vi "Disconnect Datastream Port.vi"(8 "error in (no error)":errorcluster, 11 "OXY_SCPI Reseource Out":refnum<visa-resource-name>) -> (0 "error out":errorcluster)   [LabVIEW 2020, in "OXYGEN_Datastream.lvlib"]
uses:
  OXYGEN_Datastream.lvlib
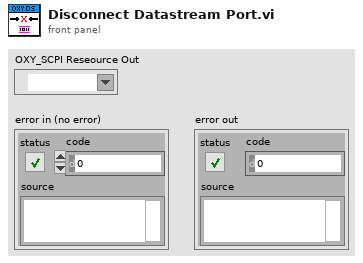
[diagram p1: front panel]
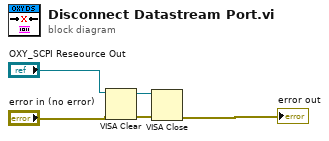
[diagram p0: block diagram]
diagram:
  n1 = VISA Clear(VISA resource name="OXY_SCPI Reseource Out", error in (no error)="error in (no error)") -> (VISA resource name out=w3:refnum<visa-resource-name>, error out=w4:errorcluster)
  n2 = VISA Close(VISA resource name=w3, error in (no error)=w4) -> (error out=→"error out":errorcluster)
